vi "Configure Bus Source (SPI-Select).vi"(6 "Shift Direction (1: MSB)":i32(ring)=1 items=["LSB", "MSB"], 7 "Polarity (0: Low)":i32(ring) items=["Low", "High"], 8 "error in (no error)":errorcluster, 9 "Select Source (9:Digital Channel 1)":u16(ring)=9 items=["Channel 1", "Channel 2", "Channel 3", "Channel 4", "Math 1", "Math 2", "Math 3", "Math 4", "Digital Channel 0", "Digital Channel 1", "Digital Channel 2", "Digital Channel 3", "Digital Channel 4", "Digital Channel 5", "Digital Channel 6", "Digital Channel 7", "Digital Channel 8", "Digital Channel 9", "Digital Channel 10", "Digital Channel 11", "Digital Channel 12", "Digital Channel 13", "Digital Channel 14", "Digital Channel 15"], 10 "BUS Number(0: Bus 1)":u8(ring) items=["Bus 1", "Bus 2", "Bus 3", "Bus 4", "Bus 5", "Bus 6", "Bus 7", "Bus 8", "Bus 9", "Bus 10", "Bus 11", "Bus 12", "Bus 13", "Bus 14", "Bus 15", "Bus 16"], 11 "VISA resource name":refnum<visa-resource-name>) -> (0 "error out":errorcluster, 3 "VISA resource name out":refnum<visa-resource-name>)   [LabVIEW 2011, in "Tektronix 7000 Series.lvlib"]
doc: "Configures SPI Bus Setting for an oscilloscope, only configures Select relative part."
uses:
  Tektronix 7000 Series.lvlib
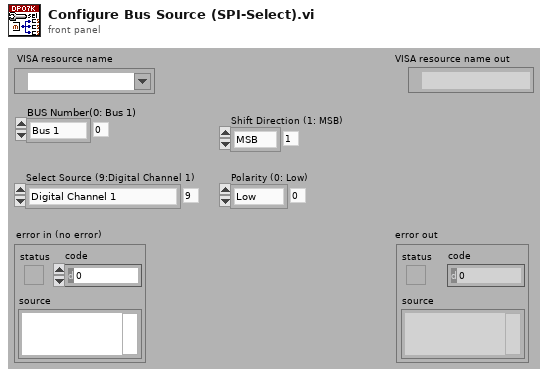
[diagram p1: front panel]
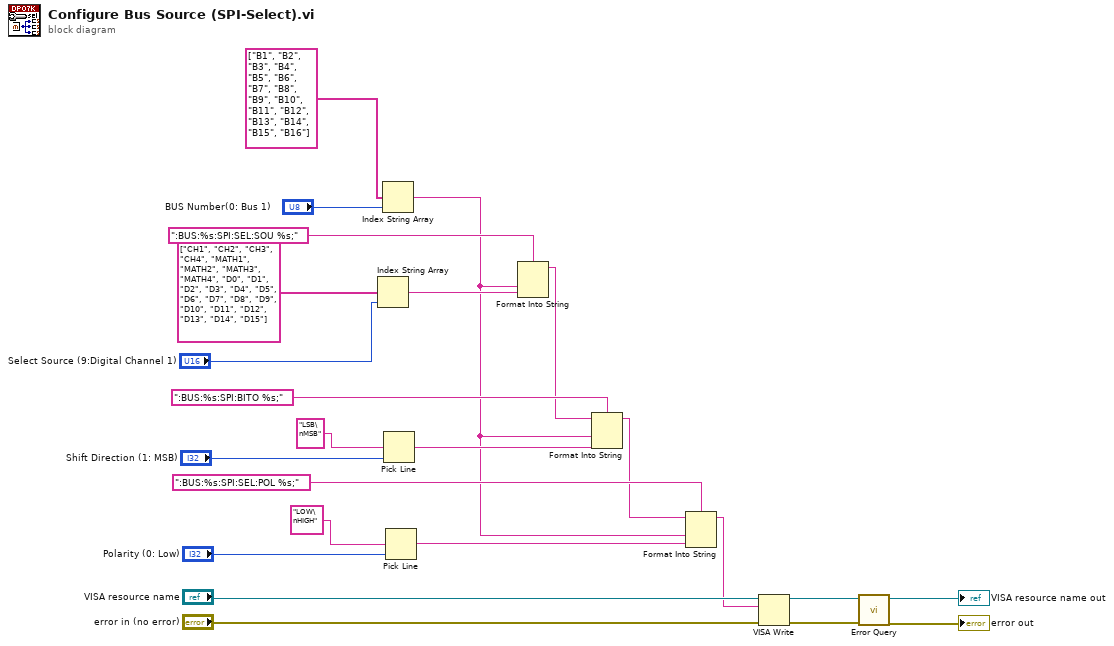
[diagram p0: block diagram]
diagram:
  n1 = Index String Array(1:"Select Source (9:Digital Channel 1)", 2:string[] ["CH1", "CH2", "CH3", "CH4", "MATH1", "MATH2", "MATH3", "MATH4", "D0", "D1", "D2", "D3", "D4", "D5", "D6", "D7", "D8", "D9", "D10", "D11", "D12", "D13", "D14", "D15"]) -> (0:w11:string)  [unwired: 1 out]
  n2 = Index String Array(1:"BUS Number(0: Bus 1)", 2:string[] ["B1", "B2", "B3", "B4", "B5", "B6", "B7", "B8", "B9", "B10", "B11", "B12", "B13", "B14", "B15", "B16"]) -> (0:w3:string)  [unwired: 1 out]
  n3 = Pick Line(multi-line string="LSB\nMSB", line index="Shift Direction (1: MSB)") -> (output string=w8:string)  [unwired: 1 out]
  n4 = Pick Line(multi-line string="LOW\nHIGH", line index="Polarity (0: Low)") -> (output string=w5:string)  [unwired: 1 out]
  n5 = Format Into String(format string=":BUS:%s:SPI:SEL:SOU %s;", w3, w11) -> (resulting string=w7:string)  [unwired: 2 in, 1 out]
  n6 = Format Into String(format string=":BUS:%s:SPI:BITO %s;", initial string=w7, w3, w8) -> (resulting string=w4:string)  [unwired: 1 in, 1 out]
  n7 = Format Into String(format string=":BUS:%s:SPI:SEL:POL %s;", initial string=w4, w3, w5) -> (resulting string=w2:string)  [unwired: 1 in, 1 out]
  n8 = VISA Write(VISA resource name="VISA resource name", write buffer=w2, error in (no error)="error in (no error)") -> (VISA resource name out=w18:refnum<visa-resource-name>, error out=w17:errorcluster)  [unwired: 1 out]
  n9 = call "Error Query.vi"("error in (no error)"=w17, "VISA resource name"=w18) -> ("error out"=→"error out":errorcluster, "VISA resource name out"=→"VISA resource name out":refnum<visa-resource-name>)  [unwired: 8 out]
